vi "Main.vi"() -> ()   [LabVIEW 2019]
uses:
  Message_Handler/typedef/Alarm_Panel.ctl
  Alarm_Panel/Channel_Temperature_Threshold.ctl
  Message_Handler/typedef/MHL_Data.ctl
  Framework/Message Queue/Enqueue Message (Single).vi
  Framework/Message Queue/Message Queue.lvlib
  Message_Handler/MHL.lvlib
  Framework/User Event - Stop/User Event - Stop.lvlib
  USB-87Pn/Module/USB-87P8_Manager.lvlib
  Logging/Data_Logger.lvlib
  Alarm_Panel/Alarm_Manager.lvlib
panel:
  out "Motor Temp Data":T1 {"[M0]" format="%#_g °C"; "[M1]" format="%#_g °C"; "[M2]" format="%#_g °C"; "[M3]" format="%#_g °C"; "[M4]" format="%#_g °C"; "[M5]" format="%#_g °C"}
  out "Bearing Temp Data":T2 {"[0]" format="%#_g °C"; "[1]" format="%#_g °C"; "[6]" format="%#_g °C"; "[7]" format="%#_g °C"; "[10]" format="%#_g °C"; "[11]" format="%#_g °C"; "[2]" format="%#_g °C"; "[3]" format="%#_g °C"; "[4]" format="%#_g °C"; "[5]" format="%#_g °C"; "[8]" format="%#_g °C"; "[9]" format="%#_g °C"; "[12]" format="%#_g °C"; "[13]" format="%#_g °C"; "[14]" format="%#_g °C"; "[15]" format="%#_g °C"}
  out "Channel (24 -31)":T3 {"Spare 7" format="%#_g °C"; "Spare 6" format="%#_g °C"; "Spare 5" format="%#_g °C"; "Spare 4" format="%#_g °C"; "Spare 3" format="%#_g °C"; "Spare 2" format="%#_g °C"; "Spare 1" format="%#_g °C"; "Spare 0" format="%#_g °C"}
  in  "Quit":bool
  in  "Motor Switch":bool
  out "Status":T4
  in  "Tab Control":T5(tab)
  out "Bearing Temperature Chart":waveform(dbl)[](graph)
  out "Motor Temperature Chart":waveform(dbl)[](graph)
  in  "Alarm Panel":T6
  # "Software version x.x www.ccsln.com"
  # "DOWTY PROPELLERS - WIND TUNNEL MOTOR TEMPERATURE MONITORING SYSTEM"
  # "Front Motor: Armature Com End"
  # "Front Motor: Field Windings"
  # "Front Motor: Armature Ctr. Brg"
  # "Rear Motor: Armature Ctr. Brg"
  # "Rear Motor: Field Windings"
  # "Rear Motor: Armature Com End"
  # "Min"
  # "Max"
  # "Alarm"
  # "Min"
  # "Max"
  # "Alarm"
  # "Min"
  # "Max"
  # "Alarm"
  # "Min"
  # "Max"
  # "Alarm"
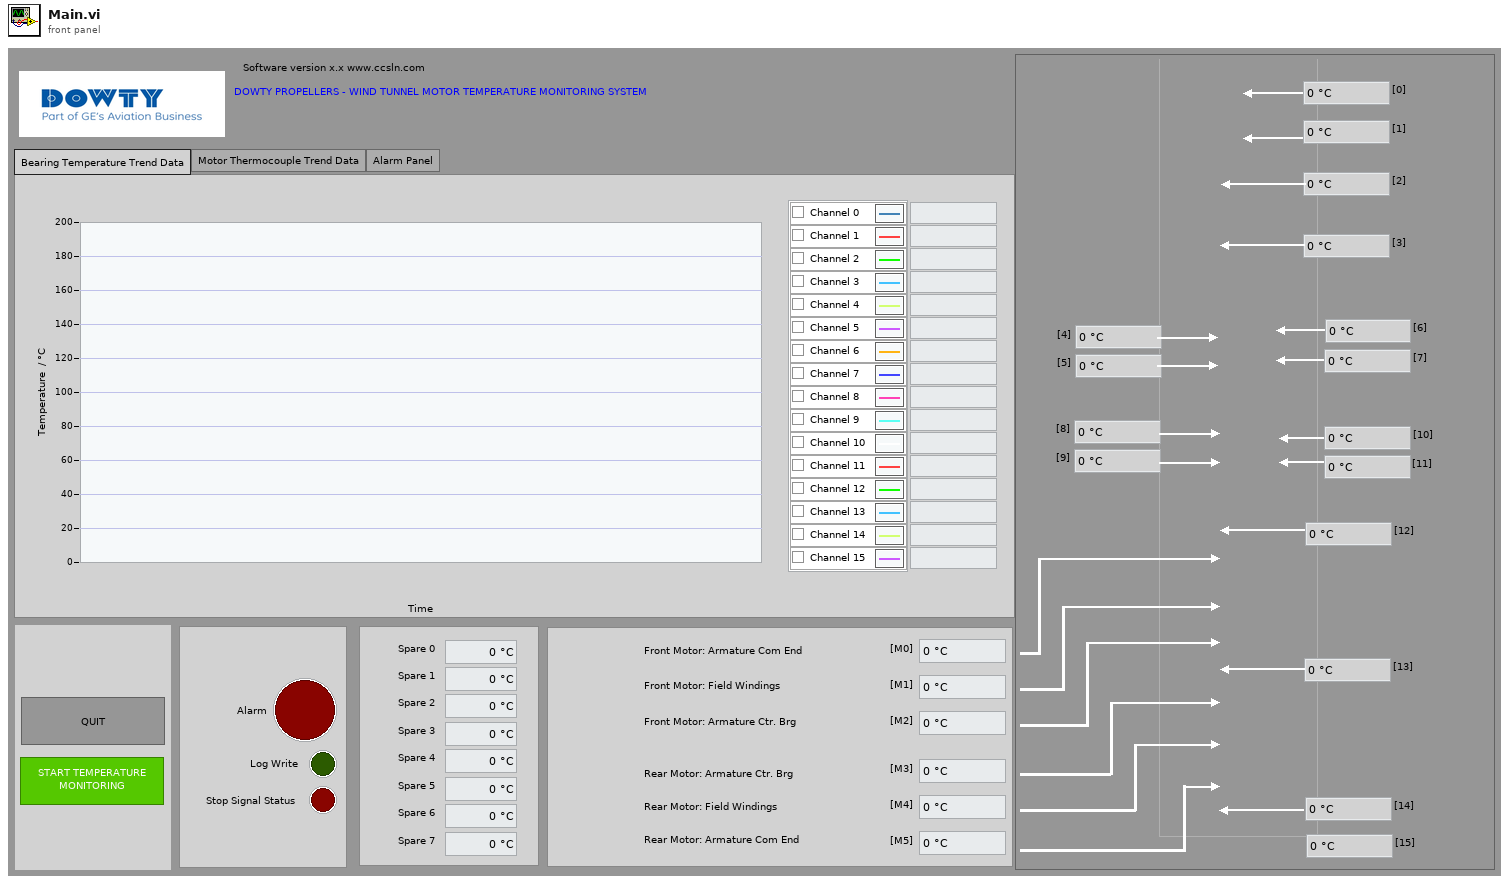
[diagram p1: front panel]
types:
  T1 = cluster{"[M0]":sgl, "[M1]":sgl, "[M2]":sgl, "[M4]":sgl, "[M5]":sgl, "[M3]":sgl}
  T2 = cluster{"[0]":sgl, "[1]":sgl, "[2]":sgl, "[3]":sgl, "[4]":sgl, "[5]":sgl, "[6]":sgl, "[7]":sgl, "[8]":sgl, "[9]":sgl, "[10]":sgl, "[11]":sgl, "[12]":sgl, "[13]":sgl, "[14]":sgl, "[15]":sgl}
  T3 = cluster{"Spare 0":dbl, "Spare 1":dbl, "Spare 2":dbl, "Spare 3":dbl, "Spare 4":dbl, "Spare 5":dbl, "Spare 6":dbl, "Spare 7":dbl}
  T4 = cluster{"Alarm":bool, "Log Write":bool, "Stop Signal Status":bool}
  T5 = enum32{"Bearing Temperature Trend Data", "Motor Thermocouple Trend Data", "Alarm Panel"}
  T6 = typedef "Alarm_Panel.ctl" = cluster{"Channel (0 - 7)":cluster{"Channel Temperature Thresholds":T7, "Channel Temperature Thresholds 2":T7, "Channel Temperature Thresholds 3":T7, "Channel Temperature Thresholds 4":T7, "Channel Temperature Thresholds 5":T7, "Channel Temperature Thresholds 6":T7, "Channel Temperature Thresholds 7":T7, "Channel Temperature Thresholds 8":T7}, "Channel (8 - 15)":cluster{"Channel Temperature Thresholds":T7, "Channel Temperature Thresholds 2":T7, "Channel Temperature Thresholds 3":T7, "Channel Temperature Thresholds 4":T7, "Channel Temperature Thresholds 5":T7, "Channel Temperature Thresholds 6":T7, "Channel Temperature Thresholds 7":T7, "Channel Temperature Thresholds 8":T7}, "Channel (16 - 23)":cluster{"Channel Temperature Thresholds":T7, "Channel Temperature Thresholds 2":T7, "Channel Temperature Thresholds 3":T7, "Channel Temperature Thresholds 4":T7, "Channel Temperature Thresholds 5":T7, "Channel Temperature Thresholds 6":T7, "Channel Temperature Thresholds 7":T7, "Channel Temperature Thresholds 8":T7}, "Channel (24 - 31)":cluster{"Channel Temperature Thresholds":T7, "Channel Temperature Thresholds 2":T7, "Channel Temperature Thresholds 3":T7, "Channel Temperature Thresholds 4":T7, "Channel Temperature Thresholds 5":T7, "Channel Temperature Thresholds 6":T7, "Channel Temperature Thresholds 7":T7, "Channel Temperature Thresholds 8":T7}}
  T7 = typedef "Channel_Temperature_Threshold.ctl" = cluster{"Min":i32, "Max":i32, "Alarm":i32, "Status":u32}
  T8 = typedef "MHL.lvlib/MHL_Data.ctl" = cluster{"Ctrl_Refs":cluster{"Quit":refnum<vi>, "Motor_Switch":refnum<vi>, "Status":refnum<vi>, "Alarm_Panel":refnum<vi>, "Bearing Temp Chart":refnum<vi>, "Motor Temp Chart":refnum<vi>, "TabCtl":refnum<vi>, "Bearing Temp Clust":refnum<vi>}, "Main_Ref":refnum<vi>}
  T9 = typedef "Message Queue.lvlib/All Message Queues.ctl" = cluster{"MHL":refnum<queue>, "USB-87P8":refnum<queue>, "Logging":refnum<queue>, "Alarm":refnum<queue>}
  T10 = cluster{"Temperature Data in[0]":sgl, "Temperature Data in[1]":sgl, "Temperature Data in[2]":sgl, "Temperature Data in[3]":sgl, "Temperature Data in[4]":sgl, "Temperature Data in[5]":sgl, "Temperature Data in[6]":sgl, "Temperature Data in[7]":sgl}
  T11 = cluster{"Temperature Data in[0]":sgl, "Temperature Data in[1]":sgl, "Temperature Data in[2]":sgl, "Temperature Data in[3]":sgl, "Temperature Data in[4]":sgl, "Temperature Data in[5]":sgl}
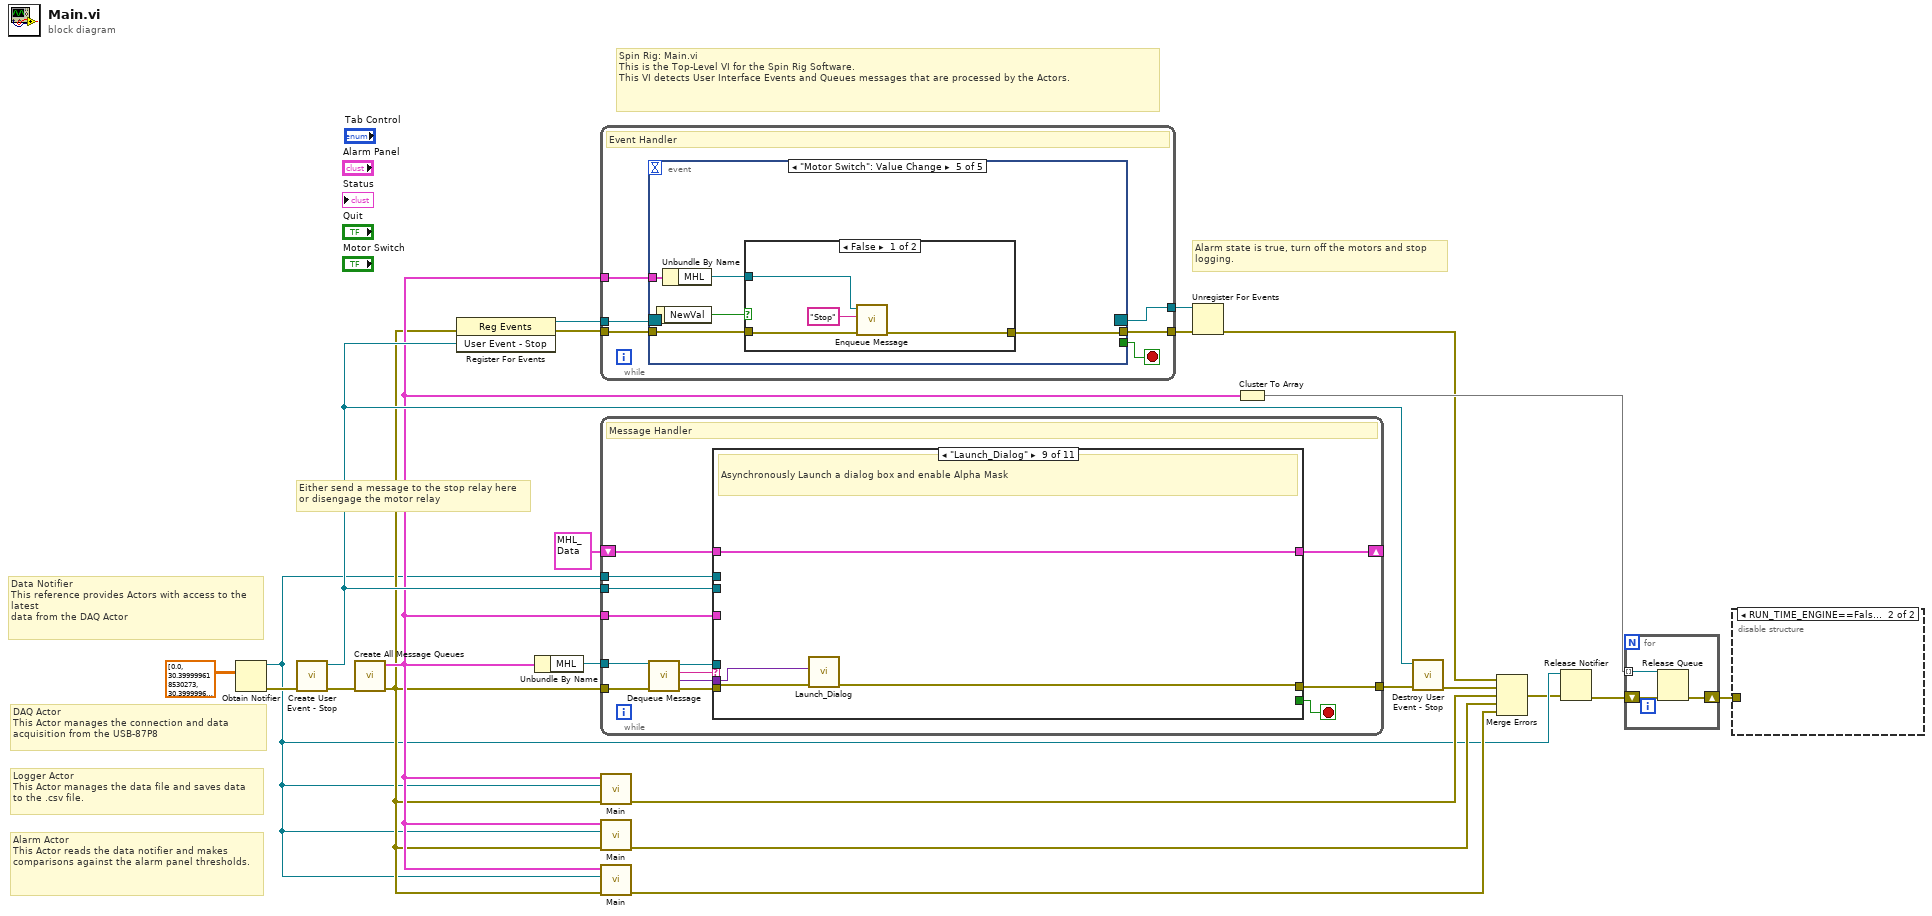
[diagram p0: block diagram]
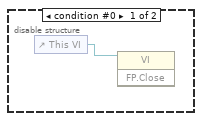
[diagram p2: hidden frame]
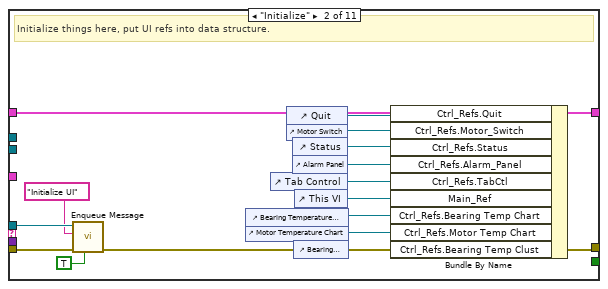
[diagram p4: hidden frame]
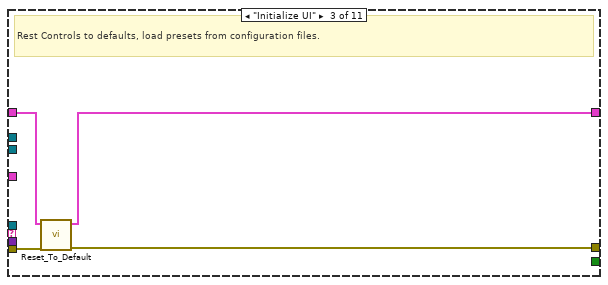
[diagram p5: hidden frame]
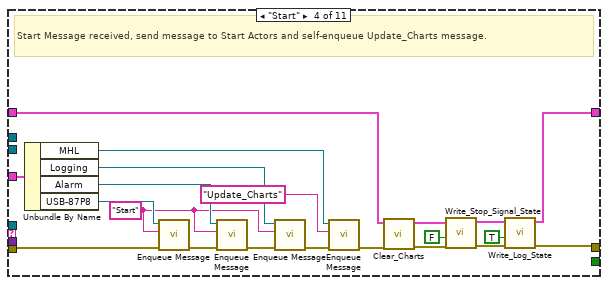
[diagram p6: hidden frame]
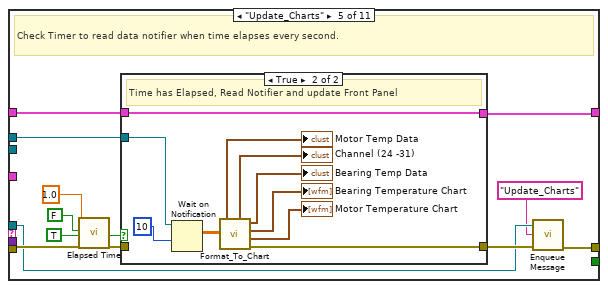
[diagram p7: hidden frame]
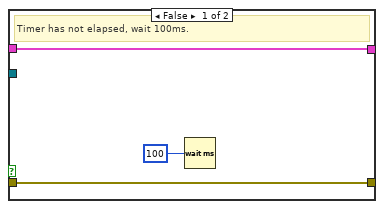
[diagram p8: hidden frame]
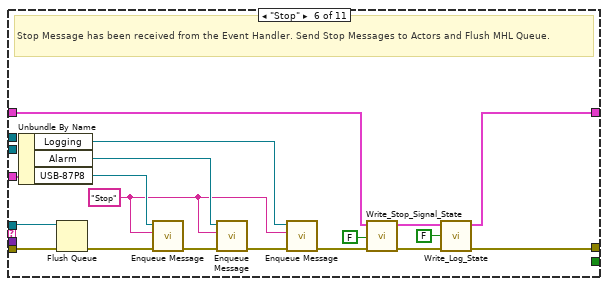
[diagram p9: hidden frame]
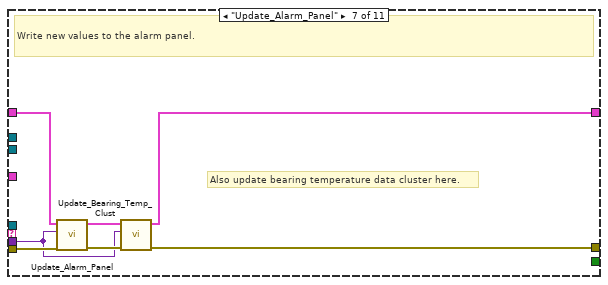
[diagram p10: hidden frame]
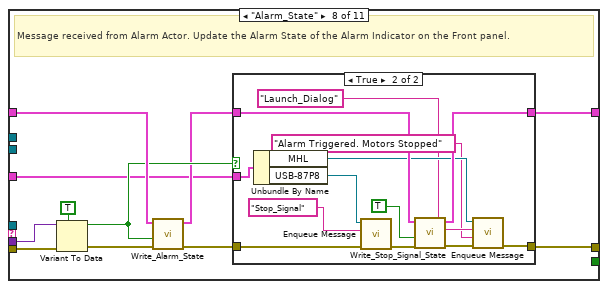
[diagram p11: hidden frame]
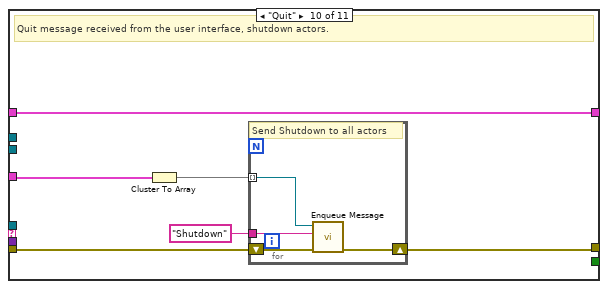
[diagram p13: hidden frame]
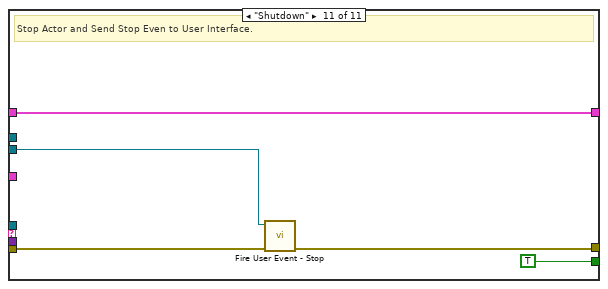
[diagram p14: hidden frame]
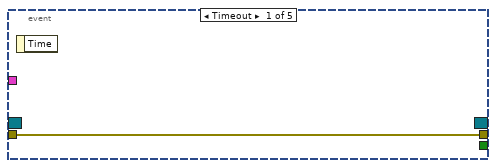
[diagram p15: hidden frame]
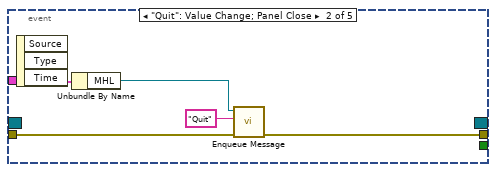
[diagram p16: hidden frame]
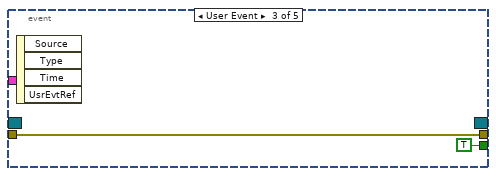
[diagram p17: hidden frame]
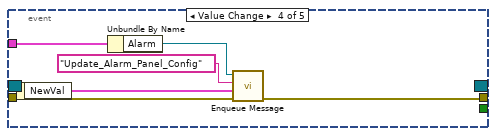
[diagram p18: hidden frame]
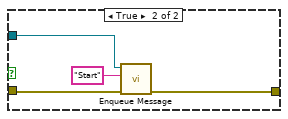
[diagram p19: hidden frame]
diagram:
  # "Either send a message to the stop relay here\nor disengage the motor relay"
  # "Alarm state is true, turn off the motors and stop\nlogging."
  # "Data Notifier\nThis reference provides Actors with access to the latest\ndata from the DAQ Actor"
  # "Alarm Actor\nThis Actor reads the data notifier and makes comparisons against the alarm panel thresholds."
  # "Logger Actor\nThis Actor manages the data file and saves data\nto the .csv file."
  # "DAQ Actor\nThis Actor manages the connection and data\nacquisition from the USB-87P8"
  # "Spin Rig: Main.vi\nThis is the Top-Level VI for the Spin Rig Software.\nThis VI detects User Interface Events and Queues messages that are processed by the Actors."
  n1 = Obtain Notifier(notification data type=sgl[][] [[0.0, 30.4, 30.4, 30.4, 30.4, 30.4, 30.3, 30.3], [35.7, 35.7, 35.7, 35.7, 35.7, 35.7, 35.7, 35.7], [31.4, 31.4, 31.4, 31.4, 31.4, 31.0, 30.8, 30.4], [32.4, 32.4, 32.4, 32.3, 32.4, 32.4, 32.5, 32.5]] ("Temperature Data")) -> (notifier out=w5:refnum<notifier>, error out=w6:errorcluster)  [unwired: 3 in, 1 out]
  n2 = call "Create User Event - Stop.vi"("error in (no error)"=w6) -> ("error out"=w21:errorcluster, "User Event - Stop"=w17:refnum<user-event>)  [unwired: 9 in]
  n3 = call "Create All Message Queues.vi"("error in (no error)"=w21) -> ("error out"=w10:errorcluster, "Message Queues out"=w11:T9)  [unwired: 9 in]
  n4 = register-events(error in=w10, w17) -> (reference out=w19:refnum<event-registration>, error out=w20:errorcluster)  [unwired: 1 in]
  n5 = Unbundle By Name(w11) -> ("MHL"=w23:refnum<queue>)
  n6 = while {
    tunnel: w11 -> [w29]
    tunnel: w20 -> [w28]
    tunnel: [w27] -> w16
    tunnel: w19 -> [w26]
    tunnel: [w24] -> w18
    stop <- w25 stop-if-true
    # "Event Handler"
    n7 = event shown="[4] \"Motor Switch\": Value Change" {
      selector: w26 -> [_ _ _ _ _]
      dyn-events: [_ _ _ _ _] -> w24
      timeout: _ -> [_ _ _ _ _]
      tunnel: w29 -> [_ w34 _ w43 w46]
      tunnel: w28 -> [w30 w35 w37 w41 w47]
      tunnel: [w30 w31 w37 w40 w44] -> w27
      tunnel: [_ _ TRUE _ _] -> w25
      event Timeout {
        n8 = event-data() -> ()  [unwired: 1 in, 1 out]
      }
      event "Quit": Value Change; Panel Close {
        n9 = event-data() -> ()  [unwired: 1 in, 3 out]
        n10 = Unbundle By Name(w34) -> ("MHL"=w33:refnum<queue>)
        n11 = call-poly "Enqueue Message.vi"("error in (no error)"=w35, "Message"="Quit", "Message Queue"=w33) -> ("error out"=w31:errorcluster)  [unwired: 7 in, 1 out]
      }
      event User Event {
        n12 = event-data() -> ()  [unwired: 1 in, 4 out]
      }
      event Value Change {
        n13 = event-data() -> ("NewVal"=w38:T6)  [unwired: 1 in]
        n14 = Unbundle By Name(w43) -> ("Alarm"=w42:refnum<queue>)
        n15 = call-poly "Enqueue Message.vi"("error in (no error)"=w41, "Message Data"=w38, "Message"="Update_Alarm_Panel_Config", "Message Queue"=w42) -> ("error out"=w40:errorcluster)  [unwired: 6 in, 1 out]
      }
      event "Motor Switch": Value Change {
        n16 = event-data() -> ("NewVal"=w48:bool)  [unwired: 1 in]
        n17 = Unbundle By Name(w46) -> ("MHL"=w45:refnum<queue>)
        n18 = case shown="False" w48 {
          tunnel: w47 -> [w51 w55]
          tunnel: w45 -> [w52 w56]
          tunnel: [w50 w54] -> w44
          frame False {
            n19 = call-poly "Enqueue Message.vi"("error in (no error)"=w51, "Message"="Stop", "Message Queue"=w52) -> ("error out"=w50:errorcluster)  [unwired: 7 in, 1 out]
          }
          frame True {
            n20 = call-poly "Enqueue Message.vi"("error in (no error)"=w55, "Message"="Start", "Message Queue"=w56) -> ("error out"=w54:errorcluster)  [unwired: 7 in, 1 out]
          }
        }
      }
    }
  }
  n21 = while {
    tunnel: w11 -> [w64]
    tunnel: w23 -> [w69]
    tunnel: w10 -> [w67]
    shift-right: [w61] -> _
    shift-left: T8 {"Ctrl_Refs"={"Quit"=refnum, "Motor_Switch"=refnum, "Status"=refnum, "Alarm_Panel"=refnum, "Bearing Temp Chart"=refnum, "Motor Temp Chart"=refnum, "TabCtl"=refnum, "Bearing Temp Clust"=refnum}, "Main_Ref"=refnum} -> [w62]
    tunnel: w17 -> [w60]
    tunnel: [w59] -> w4
    tunnel: w5 -> [w57]
    stop <- w58 stop-if-true
    # "Message Handler"
    n22 = call "Dequeue Message.vi"("error in (no error)"=w67, "Message Queue"=w69) -> ("error out"=w66:errorcluster, "Message Data"=w65:variant, "Message"=w68:string, "dup Message Queue"=w63:refnum<queue>)  [unwired: 6 in]
    n23 = case shown="\"Launch_Dialog\"" w68 {
      tunnel: w66 -> [w70 w86 w91 w110 w120 w148 w162 w174 w192 w198 w206]
      tunnel: w65 -> [_ _ _ _ _ _ w159 w173 w191 _ _]
      tunnel: w64 -> [_ _ _ w112 _ w156 _ w164 _ w195 _]
      tunnel: w63 -> [_ w87 _ _ w114 w149 _ _ _ _ _]
      tunnel: w62 -> [w71 w83 w90 w100 w124 w145 w163 w171 w193 w199 w208]
      tunnel: [w71 w82 w89 w93 w123 w141 w158 w165 w193 w199 w208] -> w61
      tunnel: w60 -> [_ _ _ _ _ _ _ _ _ _ w207]
      tunnel: [w70 w81 w88 w95 w115 w140 w157 w168 w190 w196 w205] -> w59
      tunnel: [_ _ _ _ _ _ _ _ _ _ TRUE] -> w58
      tunnel: w57 -> [_ _ _ _ w125 _ _ _ _ _ _]
      frame Default {
        # "Unknown message received."
      }
      frame "Initialize" {
        # "Initialize things here, put UI refs into data structure."
        n24 = call-poly "Enqueue Message.vi"("Priority Message? (F)"=TRUE, "error in (no error)"=w86, "Message"="Initialize UI", "Message Queue"=w87) -> ("error out"=w81:errorcluster)  [unwired: 6 in, 1 out]
        n25 = control-ref of="Bearing Temperature Chart"() -> (w75:refnum<vi>)
        n26 = control-ref of="Motor Temperature Chart"() -> (w74:refnum<vi>)
        n27 = control-ref of="Tab Control"() -> (w73:refnum<vi>)
        n28 = control-ref of="Quit"() -> (w80:refnum<vi>)
        n29 = control-ref of="Motor Switch"() -> (w79:refnum<vi>)
        n30 = control-ref of="Status"() -> (w78:refnum<vi>)
        n31 = control-ref of="Alarm Panel"() -> (w77:refnum<vi>)
        n32 = control-ref of="Bearing Temp Data"() -> (w72:refnum<vi>)
        n33 = control-ref of="This VI"() -> (w76:refnum<vi>)
        n34 = Bundle By Name(cluster=w83, "Ctrl_Refs.Quit"=w80, "Ctrl_Refs.Motor_Switch"=w79, "Ctrl_Refs.Status"=w78, "Ctrl_Refs.Alarm_Panel"=w77, "Ctrl_Refs.TabCtl"=w73, "Main_Ref"=w76, "Ctrl_Refs.Bearing Temp Chart"=w75, "Ctrl_Refs.Motor Temp Chart"=w74, "Ctrl_Refs.Bearing Temp Clust"=w72) -> (w82:T8)
      }
      frame "Initialize UI" {
        # "Rest Controls to defaults, load presets from configuration files."
        n35 = call "Reset_To_Default.vi"("error in (no error)"=w91, "MHL_Data In"=w90) -> ("error out"=w88:errorcluster, "MHL_Data Out"=w89:T8)  [unwired: 8 in]
      }
      frame "Start" {
        w105 = "Start" ("Message")
        # "Start Message received, send message to Start Actors and self-enqueue Update_Charts message."
        n36 = Unbundle By Name(w112) -> ("MHL"=w103:refnum<queue>, "Logging"=w106:refnum<queue>, "Alarm"=w108:refnum<queue>, "USB-87P8"=w111:refnum<queue>)
        n37 = call-poly "Enqueue Message.vi"("error in (no error)"=w110, "Message"=w105, "Message Queue"=w111) -> ("error out"=w109:errorcluster)  [unwired: 7 in, 1 out]
        n38 = call-poly "Enqueue Message.vi"("error in (no error)"=w109, "Message"=w105, "Message Queue"=w108) -> ("error out"=w107:errorcluster)  [unwired: 7 in, 1 out]
        n39 = call-poly "Enqueue Message.vi"("error in (no error)"=w107, "Message"=w105, "Message Queue"=w106) -> ("error out"=w104:errorcluster)  [unwired: 7 in, 1 out]
        n40 = call-poly "Enqueue Message.vi"("error in (no error)"=w104, "Message"="Update_Charts", "Message Queue"=w103) -> ("error out"=w101:errorcluster)  [unwired: 7 in, 1 out]
        n41 = call "Clear_Charts.vi"("error in (no error)"=w101, "MHL_Data In"=w100) -> ("error out"=w97:errorcluster, "MHL_Data Out"=w98:T8)  [unwired: 8 in]
        n42 = call "Write_Stop_Signal_State.vi"("error in (no error)"=w97, "Alarm_State"=FALSE, "MHL_Data In"=w98) -> ("error out"=w96:errorcluster, "MHL_Data Out"=w94:T8)  [unwired: 7 in]
        n43 = call "Write_Log_State.vi"("error in (no error)"=w96, "Alarm_State"=TRUE, "MHL_Data In"=w94) -> ("error out"=w95:errorcluster, "MHL_Data Out"=w93:T8)  [unwired: 7 in]
      }
      frame "Update_Charts" {
        # "Check Timer to read data notifier when time elapses every second."
        n44 = call "Elapsed Time"("Time Target (s)"=1.0, "Reset"=FALSE, "Auto Reset"=TRUE, "error in (no error)"=w120) -> ("Time has Elapsed"=w118:bool, "error out"=w117:errorcluster)  [unwired: 8 in, 6 out]
        n45 = case shown="True" w118 {
          tunnel: w125 -> [_ w138]
          tunnel: w124 -> [w128 w131]
          tunnel: [w128 w131] -> w123
          tunnel: [w127 w136] -> w116
          tunnel: w117 -> [w127 _]
          frame False {
            # "Timer has not elapsed, wait 100ms."
            n46 = Wait (ms)(milliseconds to wait=u32 100) -> ()  [unwired: 1 out]
          }
          frame True {
            # "Time has Elapsed, Read Notifier and update Front Panel"
            n47 = Wait on Notification(notifier=w138, timeout in ms (-1)=10) -> (notification=w137:sgl[][])  [unwired: 2 in, 3 out]
            n48 = call "Format_To_Chart.vi"("Temperature Data in"=w137) -> ("error out"=w136:errorcluster, "Motor Temperature Data"=→"Motor Temperature Chart":waveform(dbl)[], "Bearing Temperature Data"=→"Bearing Temperature Chart":waveform(dbl)[], "Bearing Temp Data"=→"Bearing Temp Data":T2, "Channel (24 - 31)"=→"Channel (24 -31)":T10, "Motor Temp Data"=→"Motor Temp Data":T11)  [unwired: 5 in]
          }
        }
        n49 = call-poly "Enqueue Message.vi"("error in (no error)"=w116, "Message"="Update_Charts", "Message Queue"=w114) -> ("error out"=w115:errorcluster)  [unwired: 7 in, 1 out]
      }
      frame "Stop" {
        w150 = "Stop" ("Message")
        # "Stop Message has been received from the Event Handler. Send Stop Messages to Actors and Flush MHL Queue."
        n50 = Unbundle By Name(w156) -> ("Logging"=w151:refnum<queue>, "Alarm"=w153:refnum<queue>, "USB-87P8"=w155:refnum<queue>)
        n51 = Flush Queue(queue=w149, error in (no error)=w148) -> (error out=w147:errorcluster)  [unwired: 2 out]
        n52 = call-poly "Enqueue Message.vi"("error in (no error)"=w147, "Message"=w150, "Message Queue"=w155) -> ("error out"=w154:errorcluster)  [unwired: 7 in, 1 out]
        n53 = call-poly "Enqueue Message.vi"("error in (no error)"=w154, "Message"=w150, "Message Queue"=w153) -> ("error out"=w152:errorcluster)  [unwired: 7 in, 1 out]
        n54 = call-poly "Enqueue Message.vi"("error in (no error)"=w152, "Message"=w150, "Message Queue"=w151) -> ("error out"=w146:errorcluster)  [unwired: 7 in, 1 out]
        n55 = call "Write_Stop_Signal_State.vi"("error in (no error)"=w146, "Alarm_State"=FALSE, "MHL_Data In"=w145) -> ("error out"=w142:errorcluster, "MHL_Data Out"=w143:T8)  [unwired: 7 in]
        n56 = call "Write_Log_State.vi"("error in (no error)"=w142, "Alarm_State"=FALSE, "MHL_Data In"=w143) -> ("error out"=w140:errorcluster, "MHL_Data Out"=w141:T8)  [unwired: 7 in]
      }
      frame "Update_Alarm_Panel" {
        # "Also update bearing temperature data cluster here."
        # "Write new values to the alarm panel."
        n57 = call "Update_Alarm_Panel.vi"("error in (no error)"=w162, "Data"=w159, "MHL_Data In"=w163) -> ("error out"=w160:errorcluster, "MHL_Data Out"=w161:T8)  [unwired: 7 in]
        n58 = call "Update_Bearing_Temp_Clust.vi"("error in (no error)"=w160, "Data In"=w159, "MHL_Data In"=w161) -> ("error out"=w157:errorcluster, "MHL_Data out"=w158:T8)  [unwired: 7 in]
      }
      frame "Alarm_State" {
        # "Message received from Alarm Actor. Update the Alarm State of the Alarm Indicator on the Front panel."
        n59 = Variant To Data(error in=w174, type=TRUE, Variant=w173) -> (data=w167:bool, error out=w170:errorcluster)
        n60 = call "Write_Alarm_State.vi"("error in (no error)"=w170, "Alarm_State"=w167, "MHL_Data In"=w171) -> ("error out"=w169:errorcluster, "MHL_Data Out"=w166:T8)  [unwired: 7 in]
        n61 = case shown="True" w167 {
          tunnel: w169 -> [w176 w189]
          tunnel: [w176 w180] -> w168
          tunnel: w166 -> [w175 w184]
          tunnel: [w175 w183] -> w165
          tunnel: w164 -> [_ w188]
          frame False {
          }
          frame True {
            n62 = Unbundle By Name(w188) -> ("MHL"=w179:refnum<queue>, "USB-87P8"=w187:refnum<queue>)
            n63 = call-poly "Enqueue Message.vi"("error in (no error)"=w189, "Message"="Stop_Signal", "Message Queue"=w187) -> ("error out"=w185:errorcluster)  [unwired: 7 in, 1 out]
            n64 = call "Write_Stop_Signal_State.vi"("error in (no error)"=w185, "Alarm_State"=TRUE, "MHL_Data In"=w184) -> ("error out"=w181:errorcluster, "MHL_Data Out"=w183:T8)  [unwired: 7 in]
            n65 = call-poly "Enqueue Message.vi"("error in (no error)"=w181, "Message Data"="Alarm Triggered. Motors Stopped" ("Message"), "Message"="Launch_Dialog", "Message Queue"=w179) -> ("error out"=w180:errorcluster)  [unwired: 6 in, 1 out]
          }
        }
      }
      frame "Launch_Dialog" {
        # "Asynchronously Launch a dialog box and enable Alpha Mask"
        n66 = call "Launch_Dialog.vi"("error in (no error)"=w192, "Dialog Text In"=w191) -> ("error out"=w190:errorcluster)  [unwired: 9 in]
      }
      frame "Quit" {
        # "Quit message received from the user interface, shutdown actors."
        n67 = Cluster To Array(cluster=w195) -> (array=w194:refnum<queue>[])
        n68 = for {
          tunnel: "Shutdown" ("Message") -> [w202]
          shift-right: [w201] -> w196
          shift-left: w198 -> [w203]
          tunnel: w194 -> [w200] mode=indexing
          # "Send Shutdown to all actors"
          n69 = call-poly "Enqueue Message.vi"("error in (no error)"=w203, "Message"=w202, "Message Queue"=w200) -> ("error out"=w201:errorcluster)  [unwired: 7 in, 1 out]
        }
      }
      frame "Shutdown" {
        # "Stop Actor and Send Stop Even to User Interface."
        n70 = call "Fire User Event - Stop.vi"("error in (no error)"=w206, "User Event - Stop"=w207) -> ("error out"=w205:errorcluster)  [unwired: 9 in]
      }
    }
  }
  n71 = call "Main.vi"("error in (no error)"=w10, "Temperature_Notifier"=w5, "Message Queues"=w11) -> ("error out"=w12:errorcluster)  [unwired: 8 in]
  n72 = call "Main.vi"("error in (no error)"=w10, "Temperature_Notifier"=w5, "Message Queues"=w11) -> ("error out"=w9:errorcluster)  [unwired: 8 in]
  n73 = call "Main.vi"("error in (no error)"=w10, "Temperature_Notifier"=w5, "Message Queues"=w11) -> ("error out"=w8:errorcluster)  [unwired: 8 in]
  n74 = Unregister For Events(event registration refnum=w18, error in=w16) -> (error out=w13:errorcluster)
  n75 = Cluster To Array(cluster=w11) -> (array=w15:refnum<queue>[])
  n76 = call "Destroy User Event - Stop.vi"("error in (no error)"=w4, "User Event - Stop"=w17) -> ("error out"=w14:errorcluster)  [unwired: 9 in]
  n77 = Merge Errors(w13, w14, w12, w9, w8) -> (w3:errorcluster)
  n78 = Release Notifier(notifier=w5, error in (no error)=w3) -> (error out=w2:errorcluster)  [unwired: 1 in, 2 out]
  n79 = for {
    tunnel: w15 -> [w211] mode=indexing
    shift-right: [w209] -> w1
    shift-left: w2 -> [w210]
    n80 = Release Queue(queue=w211, error in (no error)=w210) -> (error out=w209:errorcluster)  [unwired: 1 in, 2 out]
  }
  n81 = disable-structure shown="RUN_TIME_ENGINE==False" {
    disable-tunnel: w1 -> [_ _]
    frame condition #0 {
      n82 = control-ref of="This VI"() -> (w212:refnum<vi>)
      n83 = invoke class="VI" method="FP.Close"(reference=w212) -> ()  [unwired: 2 in, 3 out]
    }
    frame condition #1 (active) {
    }
  }
